vi "StringChannelDIGSelector.vi"(7 "ComboBoxREF":refnum<vi>, 8 "error in (no error)":errorcluster, 11 "input string":string="1") -> (0 "error out":errorcluster, 3 "trigger source (dig)":T1="VAL_RTSI_0" caption="trigger source (RTSI 0)")   [LabVIEW 2011]
uses:
  niScope trigger source digital.ctl
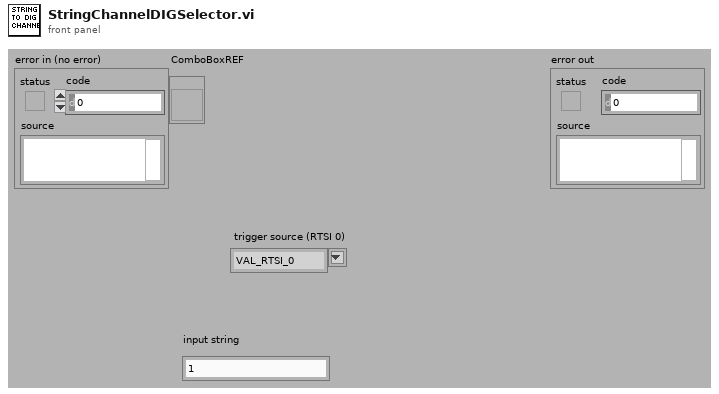
[diagram p1: front panel]
types:
  T1 = typedef "niScope trigger source digital.ctl" = string
  T2 = typedef "LVComboBoxStrsAndValuesArrayTypeDef.ctl" = cluster{"String":string, "Value":string}[]
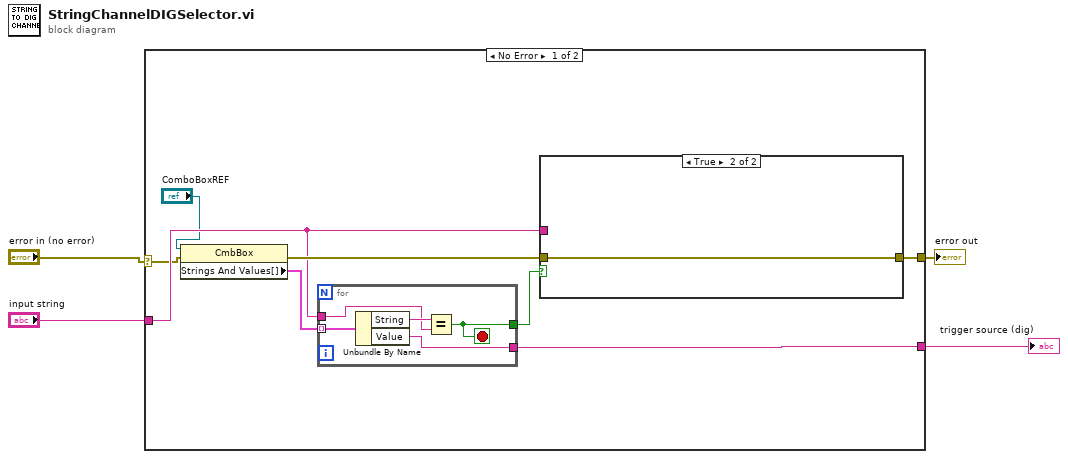
[diagram p0: block diagram]
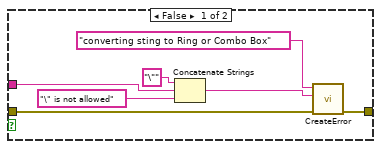
[diagram p2: hidden frame]
diagram:
  n1 = case shown="No Error" "error in (no error)" {
    selector: "error in (no error)" -> [w5 w26]
    tunnel: [w11 w27] -> w4
    tunnel: "input string" -> [w8 w27]
    tunnel: [w7 w26] -> w2
    frame No Error {
      n2 = property class="CmbBox"(reference="ComboBoxREF", error in=w5) -> (error out=w9:errorcluster, "Strings And Values[]"=w12:T2)  [unwired: 1 out]
      n3 = for {
        tunnel: w12 -> [w25] mode=indexing
        tunnel: w8 -> [w23]
        tunnel: [w22] -> w11
        tunnel: [w21] -> w10
        stop <- w21 stop-if-true
        n4 = Unbundle By Name(w25) -> ("String"=w24:string, "Value"=w22:string)
        n5 = Equal?(x=w24, y=w23) -> (x = y?=w21:bool)
      }
      n6 = case shown="True" w10 {
        tunnel: w9 -> [w19 w20]
        tunnel: [w18 w20] -> w7
        tunnel: w8 -> [w16 _]
        frame False {
          n7 = Concatenate Strings("\"" ("string"), w16, "\" is not allowed" ("string")) -> (w13:string)
          n8 = call "CreateError.vi"("user error in"=w19, "error message (\"\")"=w13, "command"="converting sting to Ring or Combo Box") -> ("user error  out"=w18:errorcluster)  [unwired: 8 in]
        }
        frame True {
        }
      }
    }
    frame Error {
    }
  }
  "trigger source (dig)" <- w4
  "error out" <- w2
